vi "Implement Publication Policy.vi"(5 "Last Published Value":variant, 7 "Last Published Time":timestamp, 9 "New Value Time":timestamp, 10 "New Value":variant, 11 "PublicationPolicy":refnum<class "IPublicationPolicy.lvclass">) -> (0 "error out (Reject Publication)":errorcluster, 2 "Value to Publish":variant)   [LabVIEW 2018, in "MVA Framework.lvlib" / "IMediator.lvlib" / "IPublicationPolicy.lvclass"]
doc: "此方法决定是否发送或以其他方式处理新数据值。该策略由订阅者设置和维护。Topic Actor不知道任何策略细节，它只是将新值传入。如果此方法内部出现故障，Topic Acton必须假设侦听器不再有效（死亡/不可恢复），并应将其从订阅服务器列表中删除。"
uses:
  IPublicationPolicy.lvclass
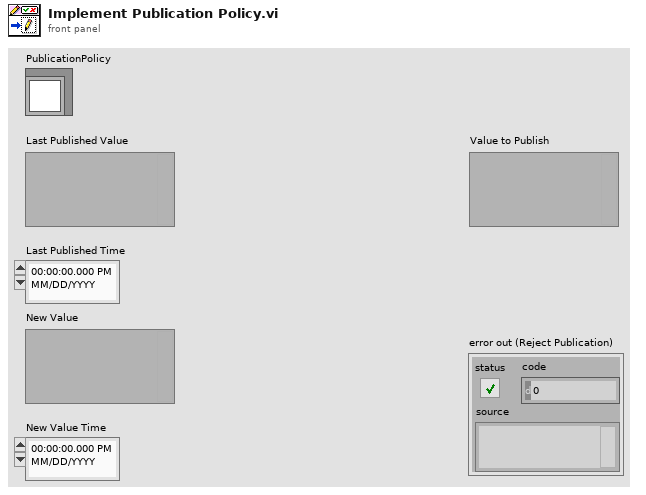
[diagram p1: front panel]
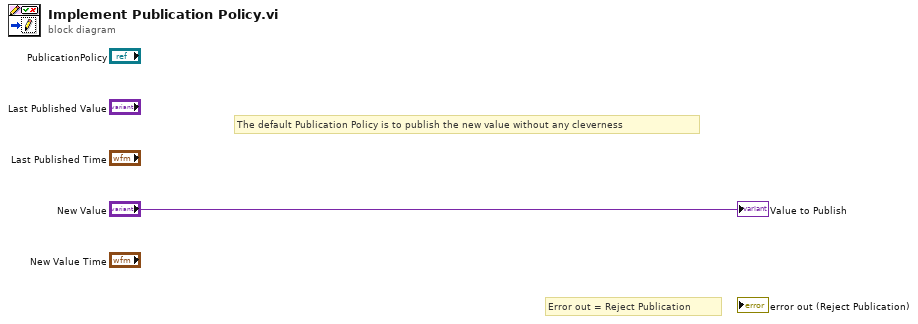
[diagram p0: block diagram]
diagram:
  # "The default Publication Policy is to publish the new value without any cleverness"
  # "Error out = Reject Publication"
  "Value to Publish" <- "New Value"
